vi "sv_Compute Swept FRF.vi"(7 "swept sine measurements":T1 {"scaled response magnitude" format="%.3f"; "Harm[]" format="%.2f"; "THD" format="%.2f"; "Im [response]" format="%.2f"; "Re [response]" format="%.2f"; "Im [stimulus]" format="%.2f"; "Re [stimulus]" format="%.2f"; "RMS response" format="%.2f"; "RMS stimulus" format="%.2f"}, 8 "error in (no error)":errorcluster) -> (0 "error out":errorcluster, 1 "phase (radian)":dbl[](array[numeric]) format="%.2f", 2 "magnitude":dbl[](array[numeric]) format="%.2f", 5 "dup swept sine measurements":T1 {"scaled response magnitude" format="%.3f"; "Harm[]" format="%.2f"; "THD" format="%.2f"; "Im [response]" format="%.2f"; "Re [response]" format="%.2f"; "Im [stimulus]" format="%.2f"; "Re [stimulus]" format="%.2f"; "RMS response" format="%.2f"; "RMS stimulus" format="%.2f"}, 6 "nyquist plot":cluster{"Re [FRF]":dbl[], "Im [FRF]":dbl[]} {"Im [FRF]" format="%.2f"; "Re [FRF]" format="%.2f"})   [LabVIEW 2017, in "SoundVib_SweptSine.lvlib"]
uses:
  <vilib>/addons/Sound and Vibration/svt_Swept Sine/SoundVib_SweptSine.lvlib
  <vilib>/addons/Sound and Vibration/svt_Swept Sine/subVIs/sv_Swept Sine Measurements.ctl
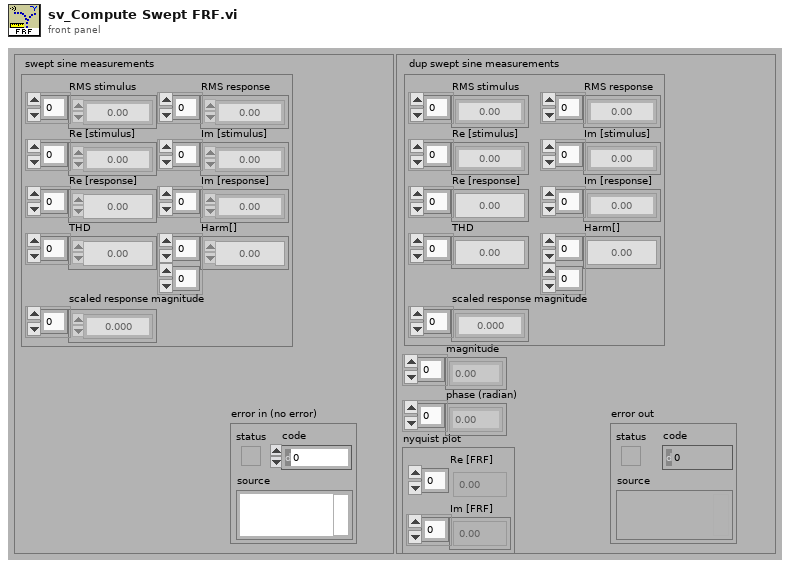
[diagram p1: front panel]
types:
  T1 = typedef "SoundVib_SweptSine.lvlib/sv_Swept Sine Measurements.ctl" = cluster{"RMS stimulus":dbl[], "RMS response":dbl[], "Re [stimulus]":dbl[], "Im [stimulus]":dbl[], "Re [response]":dbl[], "Im [response]":dbl[], "THD":dbl[], "Harm[]":dbl[][], "scaled response magnitude":dbl[]}
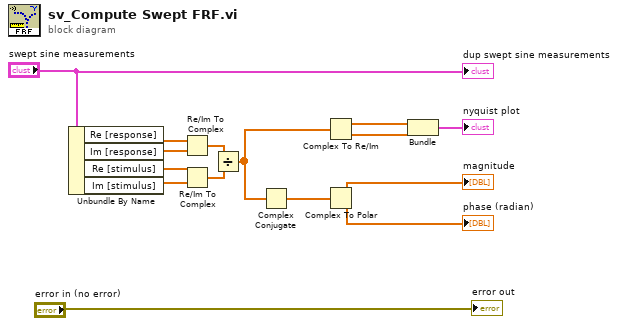
[diagram p0: block diagram]
diagram:
  n1 = Unbundle By Name("swept sine measurements") -> ("Re [response]"=w8:dbl[], "Im [response]"=w9:dbl[], "Re [stimulus]"=w10:dbl[], "Im [stimulus]"=w11:dbl[])
  n2 = Re/Im To Complex(1:w9, 2:w8) -> (0:w5:cdb[])
  n3 = Re/Im To Complex(1:w11, 2:w10) -> (0:w4:cdb[])
  n4 = Divide(x=w5, y=w4) -> (x/y=w1:cdb[])
  n5 = Complex Conjugate(1:w1) -> (0:w2:cdb[])
  n6 = Complex To Re/Im(x + iy=w1) -> (x=w13:dbl[], y=w14:dbl[])
  n7 = Complex To Polar(r * e^(i*theta)=w2) -> (r=→"magnitude":dbl[], theta=→"phase (radian)":dbl[])
  n8 = Bundle(w13, w14) -> (→"nyquist plot":cluster{dbl[], dbl[]})  [unwired: 1 in]
  "dup swept sine measurements" <- "swept sine measurements"
  "error out" <- "error in (no error)"
